vi "写入Function.vi"(8 "error in (no error)":errorcluster caption="错误输入（无错误）", 10 "Function":T1, 11 "DP输入":refnum<class "DP.lvclass">) -> (0 "error out":errorcluster caption="错误输出", 3 "DP输出":refnum<class "DP.lvclass">)   [LabVIEW 2020, in "DP.lvlib" / "DP.lvclass"]
uses:
  DP.lvclass
  Function.ctl
  DP.lvclass/DP.ctl
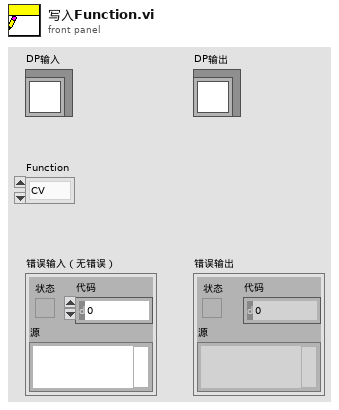
[diagram p1: front panel]
types:
  T1 = typedef "DP.lvlib/DP.lvclass/Function.ctl" = enum16{"CV", "CC"}
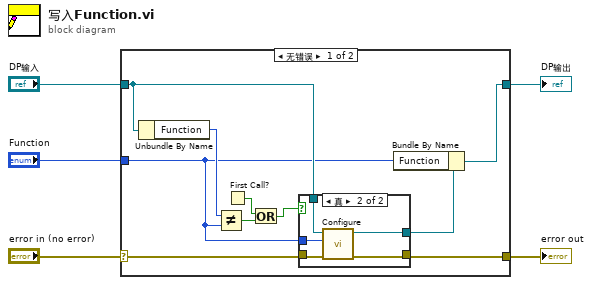
[diagram p0: block diagram]
diagram:
  n1 = case shown="无错误" "error in (no error)" {
    selector: "error in (no error)" -> [w13 w23]
    tunnel: [w12 w23] -> w1
    tunnel: [w15 w24] -> w4
    tunnel: "DP输入" -> [w11 w24]
    tunnel: "Function" -> [w9 _]
    frame No Error {
      n2 = Unbundle By Name(w11) -> ("Function"=w10:T1)
      n3 = Not Equal?(x=w10, y=w9) -> (x != y?=w8:bool)
      n4 = First Call?() -> (First Call?: T/F=w6:bool)
      n5 = Or(x=w6, y=w8) -> (x .or. y?=w7:bool)
      n6 = case shown="真" w7 {
        tunnel: [w17 w22] -> w14
        tunnel: w13 -> [w16 w21]
        tunnel: [w16 w20] -> w12
        tunnel: w11 -> [w17 w19]
        tunnel: w9 -> [_ w18]
        frame False {
        }
        frame True {
          n7 = call-dynamic "Configure.vi"("error in (no error)"=w21, "Function"=w18, "DP 输入"=w19) -> ("error out"=w20:errorcluster, "DP 输出"=w22:refnum<class "DP.lvclass">)  [unwired: 7 in]
        }
      }
      n8 = Bundle By Name(cluster=w14, "Function"=w9) -> (w15:refnum<class "DP.lvclass">)
    }
    frame Error {
    }
  }
  "error out" <- w1
  "DP输出" <- w4
